vi "Update Report Previous RUNs.vi"(8 "error in (no error)":errorcluster, 10 "Previous RUN outcome":string, 11 "Monkey in":refnum<class "Monkey.lvclass">) -> (0 "error out":errorcluster, 3 "Monkey out":refnum<class "Monkey.lvclass">)   [LabVIEW 2020, in "Monkey.lvlib" / "Monkey.lvclass"]
doc: "Add a timestamped line to the report message with the final result of the script"
uses:
  Monkey.lvclass
  C:/Users/marco/Documents/GitHub_Lab/TALOS/talos/Father of all uServices/Father of all uServices/Father of all uServices.lvclass
  Father of all uServices/Father of all uServices/Father of all uServices.lvclass/Father of all uServices.ctl
  Ancestor/Ancestor/Ancestor.lvclass/Ancestor.ctl
  Father of all uServices/Father of all uServices/Children Methods/Update GUI.vi
  Support VIs/Substitute Error.vi
  Support VIs/Generate Error.vi
  FGV/Error Memory/Get Error Description.vi
  Support VIs/Get PC name.vi
  Ancestor/Ancestor/Read ID.vi
  Support VIs/Get Class Name.vi
  <vilib>/Utility/error.llb/Clear Errors.vi
  FGV/Error Memory/Error Memory Core.vi
  <vilib>/AdvancedString/Delimited String to 1D String Array.vi
  Support VIs/Circus Root Path.vi
  FGV/Error Memory/Error Crt Lvl checker.vi
  FGV/Error Memory/Error Memory Core.vi/40c8088d-b597-4017-91af-faa98e00292e.vi
  FGV/Error Memory/Error Memory Core.vi/d4a3ab98-063c-4e44-b43d-fbdcfe6c2be2.vi
  Father of all uServices/Father of all uServices/Children Methods/Get GUI Item Value - String.vi
  Father of all uServices/Father of all uServices/Multiline string updater.vi
  Support VIs/Global Memory.vi
  <vilib>/Utility/LVClass/Get LV Class Name.vi
  Support VIs/Is in Packed Library.vi
  Support VIs/TALOS Root path.vi
  Support VIs/Read CSV worksheet.vi
  Support VIs/Global Constants.vi
  <vilib>/Utility/error.llb/General Error Handler.vi
  Support VIs/Error Log.vi
  Run Utilities/Run Block/Run Block.lvclass
  Ancestor/Ancestor/Ancestor.lvclass
  <vilib>/Comparison/Equal/Equal Functor/Equal Functor.lvclass
  Father of all uServices/Father of all uServices/Father of all uServices.lvclass
  TALOS.lvlib
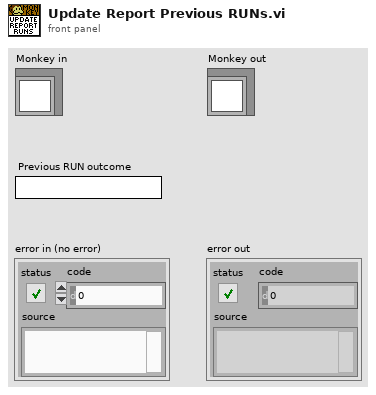
[diagram p1: front panel]
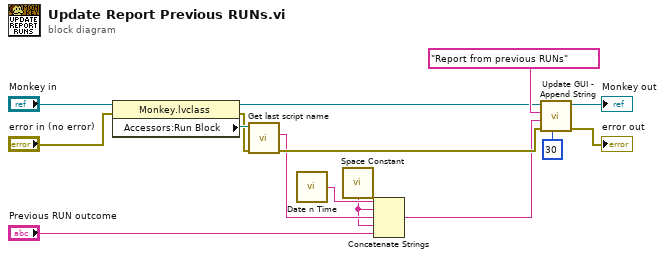
[diagram p0: block diagram]
diagram:
  n1 = property class="Monkey.lvclass"(reference="Monkey in", error in="error in (no error)") -> (reference out=w3:refnum<class "Monkey.lvclass">, error out=w4:errorcluster, "Accessors:Run Block"=w6:refnum<class "Run Block.lvclass">)
  n2 = call-dynamic "Get last script name.vi"("error in (no error)"=w4, "Run Block in"=w6) -> ("error out"=w15:errorcluster, "Last script name"=w5:string)  [unwired: 7 in, 1 out]
  n3 = call "Date n Time.vi"() -> ("Date & Time"=w9:string)  [unwired: 5 in]
  n4 = call <vilib>:"Space Constant.vi"() -> ("String"=w2:string)
  n5 = Concatenate Strings(w9, w2, w5, w2, "Previous RUN outcome") -> (w10:string)
  n6 = call "Update GUI - Append String.vi"("Lines to keep"=u8 30, "error in (no error)"=w15, "String"=w10, "GUI Item Name"="Report from previous RUNs", "Father of all uServices in"=w3) -> ("error out"=→"error out":errorcluster, "Father of all uServices out"=→"Monkey out":refnum<class "Monkey.lvclass">)  [unwired: 5 in]
